vi "Compute Depth Image.vi"() -> ()   [LabVIEW 2014]
doc: "This example demonstrates the binocular stereo vision algorithms installed with NI Vision Development Module."
uses:
  <vilib>/vision/NI_Vision_Development_Module.lvlib
panel:
  out "SGBM Time":dbl caption="Time to Compute Depth Image"
  out "SGBM Time":dbl caption="Time to Compute Depth Image"
  out "SGBM Depth":dbl caption="Depth"
  out "Depth - Block Matching Algorithm":sgl[][](graph)
  out "Depth - Semi Global Block Matching Algorithm":sgl[][](graph)
  out "BM Depth":dbl caption="Depth"
  in  "Stop":bool
  in  "Select Image":i32(slide) min=0 max=5 step=1 scale=0.0..4.0
  out "Calibrating":bool=TRUE
  out "Right Image":T1(plugin-control)
  out "Left Image":T1(plugin-control)
  # "Overview: Demonstrate how to calibrate a stereo vision system and compute a depth image.\nRequirements: Vision Development Module.\nNote: This example does not run on LabVIEW Real Time\nInstructions:\n1. Run the VI.\n2. Select an image with the Select Image control\n3. Mouse over any image to view the depth at the mouse location."
  # "in"
  # "in"
  # "in"
  # "in"
  # "Mouse over the image to view the depth."
  # "inches"
  # "inches"
  # "Mouse over the image to view the depth."
  # "ms"
  # "ms"
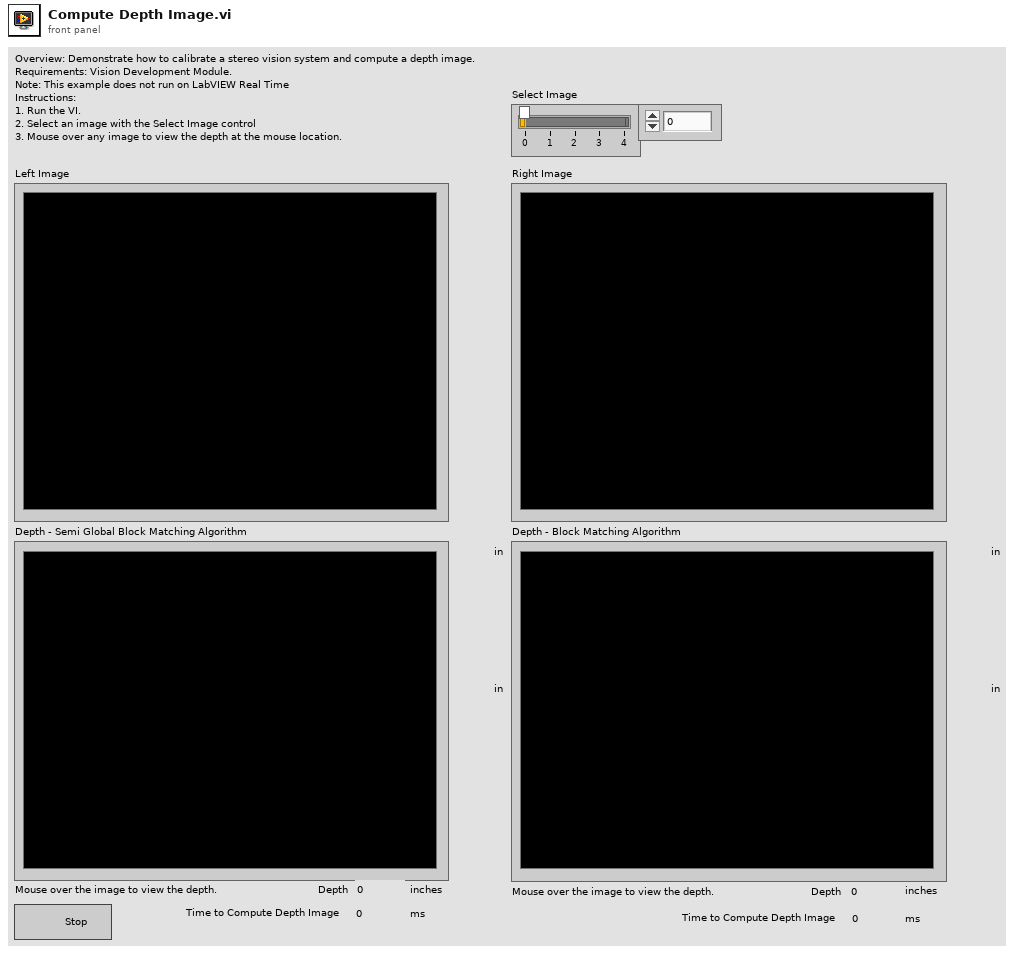
[diagram p1: front panel]
types:
  T1 = typedef "IMAQ Image.ctl" = refnum<image>
  T2 = cluster{"Number of Disparity":dbl, "Number of Disparity":dbl}
  T3 = typedef "Calibration Reference Points.ctl" = cluster{"Pixel Coordinates":cluster{"X":dbl, "Y":dbl}[], "Real World Coordinates":cluster{"X":dbl, "Y":dbl}[], "Unit":T4, "Image Size":cluster{"X":u32, "Y":u32}}
  T4 = typedef "Image Unit" = enum32{"Undefined", "Angström", "Micrometer", "Millimeter", "Centimeter", "Meter", "Kilometer", "Microinch", "Inch", "Feet", "Nautical miles", "Standard miles", "Steps"}
  T5 = typedef "IMAQ Binocular Stereo Session.ctl" = refnum<k1>
  T6 = typedef "Image Type" = u32
  T7 = cluster{"Method":u16, "Window Size":dbl, "Minimum Disparity":dbl, "Number of Disparity":dbl, "Left - Right Check":dbl, "Subpixel":bool, "Invalid Disparity Replace Value":dbl}
  T8 = cluster{"Filter Type":u16, "Filter Size":dbl, "Filter Cap":dbl}
  T9 = cluster{"Texture Threshold":dbl, "Uniqueness Ratio":dbl, "Speckle Window Size":dbl, "Speckle Range":dbl}
  T10 = cluster{"Method":u16, "Window Size":dbl, "Minimum Disparity":dbl, "Number of Disparity":dbl, "P1":dbl, "P2":dbl, "Full DP":bool, "Max Left Right Disparity":dbl, "Subpixel":bool, "Invalid Disparity Replace Value":dbl}
  T11 = typedef "LVPoint32TypeDef.ctl" = cluster{"Horizontal":i32, "Vertical":i32}
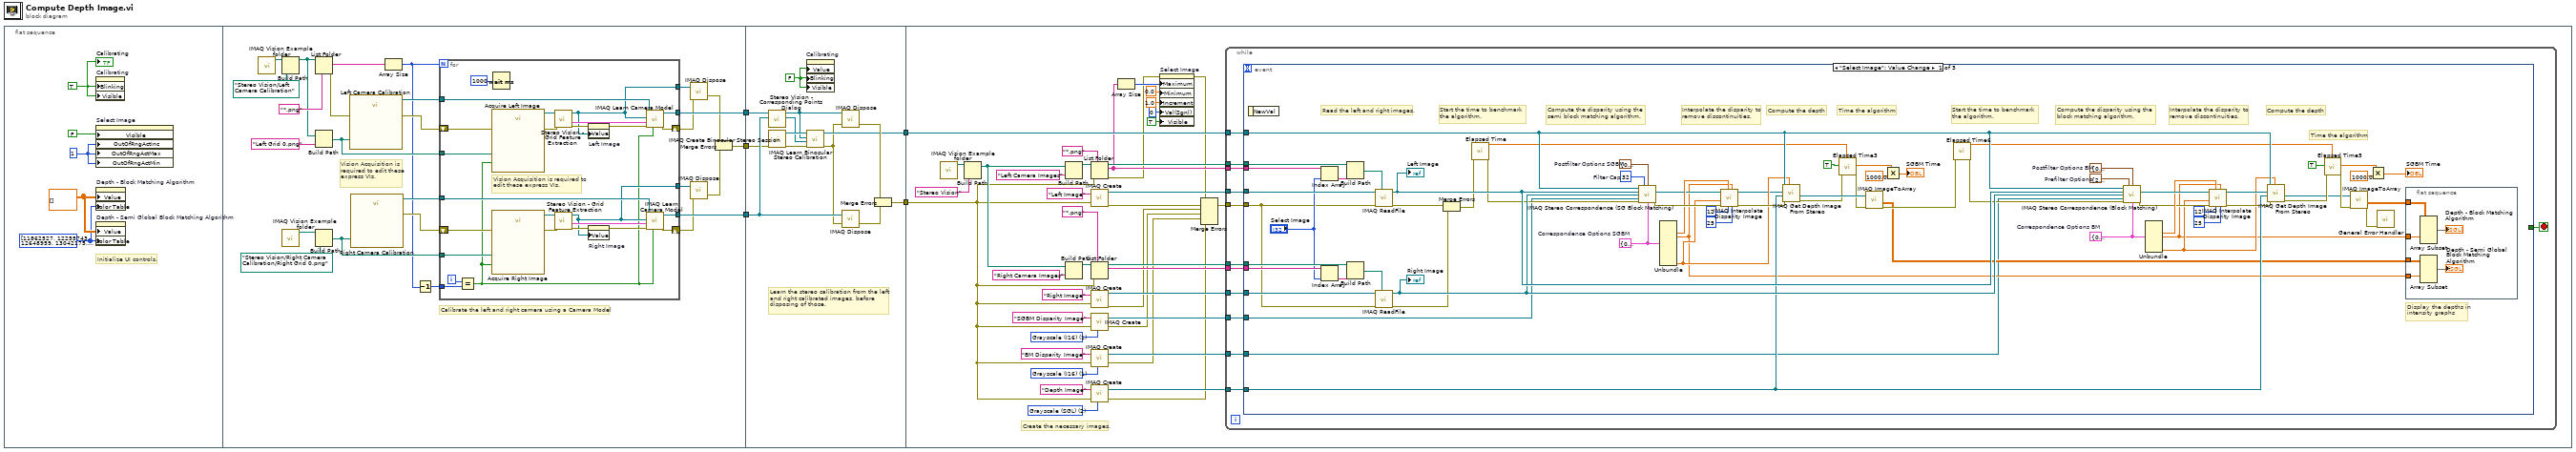
[diagram p0: block diagram]
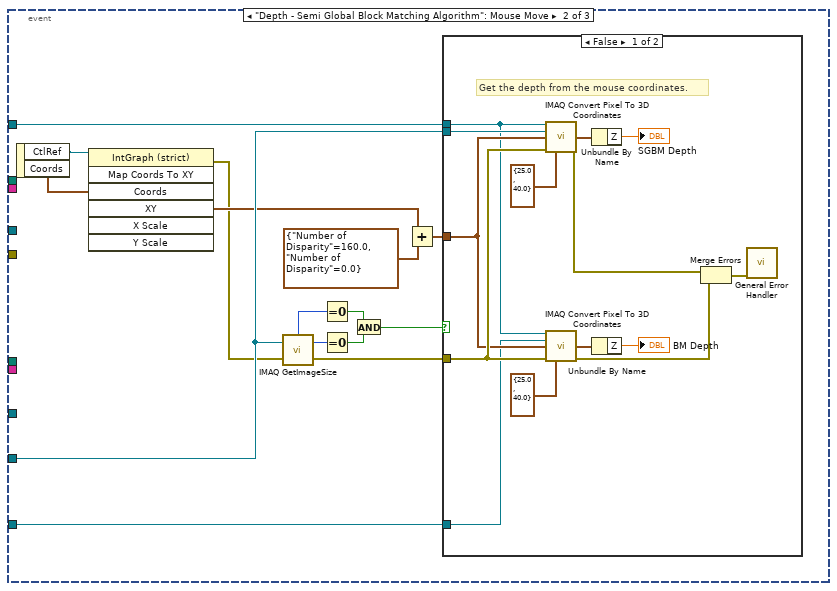
[diagram p2: hidden frame]
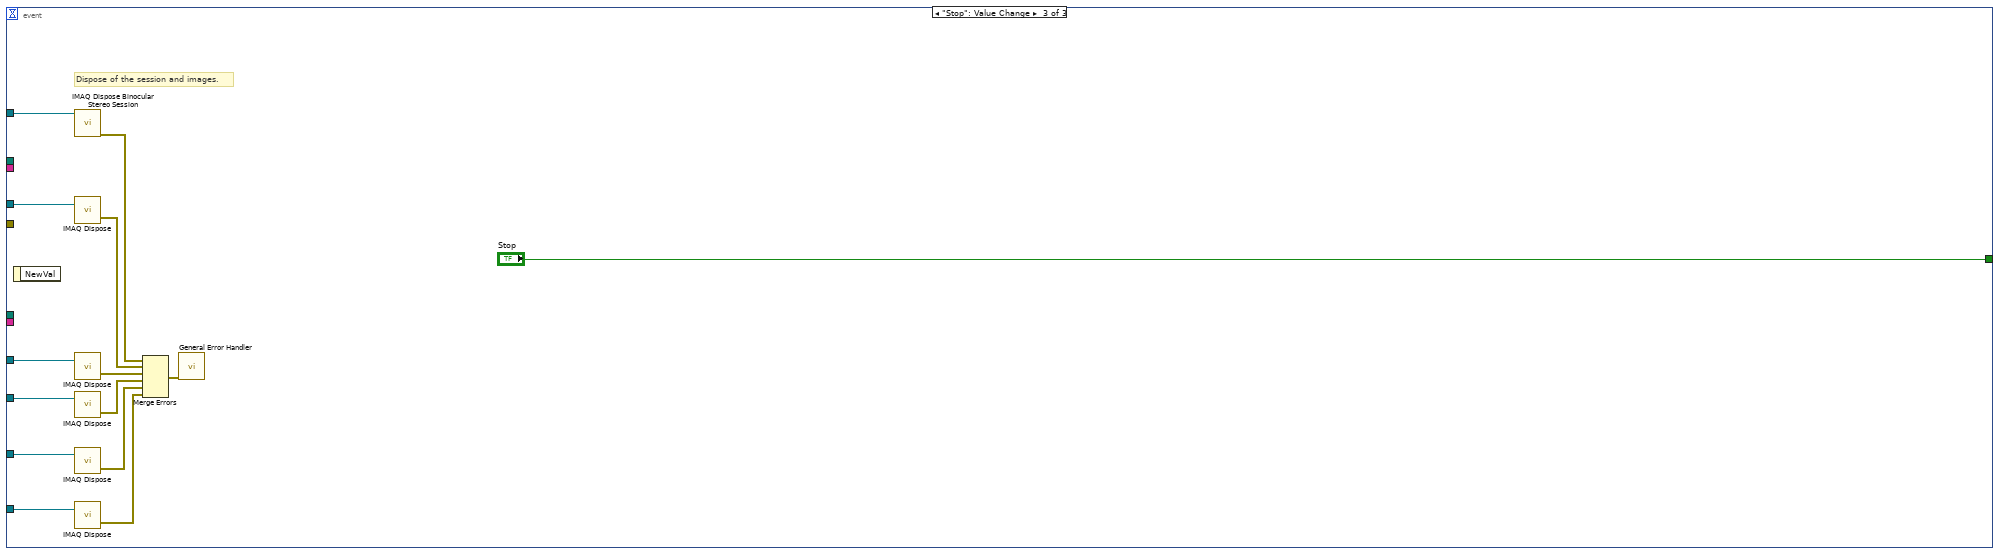
[diagram p4: hidden frame]
diagram:
  n1 = flat-sequence {
    tunnel: [w33] -> w5
    tunnel: [w36] -> w4
    tunnel: [w32] -> w2
    tunnel: w5 -> [w72]
    tunnel: w4 -> [w71]
    tunnel: [w64] -> w3
    tunnel: w2 -> [w68]
    tunnel: [w65] -> w1
    tunnel: w3 -> [w99]
    tunnel: w1 -> [w79]
    frame #0 {
      w6 = u32[] [11862527, 12255743, 12648959, 13042175, 13435391, 13828607, 14221823, 14615039, 15008255, 15401471, 15794687, 16187903, 16581119, 16712189, 16712183, 16712177, 16712171, 16712165, 16712159, 16712153, 16712147, 16712141, 16712135, 16712129, 16712123, 16712117, 16712111, 16712105, 16712099, 16712093, 16712087, 16712081, 16712075, 16712069, 16712063, 16712057, 16712051, 16712045, 16712039, 16712033, 16712027, 16712021, 16712015, 16712009, 16712003, 16711997, 16711991, 16711985, 16711979, 16711973, 16711967, 16711961, 16711955, 16711949, 16711943, 16711937, 16711937, 16713473, 16715009, 16716545, 16718081, 16719617, 16721153, 16722689, 16724225, 16725761, 16727297, 16728833, 16730369, 16731905, 16733441, 16734977, 16736513, 16738049, 16739585, 16741121, 16742657, 16744193, 16745729, 16747265, 16748801, 16750337, 16751873, 16753409, 16754945, 16756481, 16758017, 16759553, 16761089, 16762625, 16765697, 16767233, 16768769, 16770305, 16771841, 16773377, 16774913, 16776449, 16645889, 16252673, 15859457, 15466241, 15073025, 14679809, 14286593, 13893377, 13500161, 13106945, 12713729, 12320513, 11927297, 11534081, 11140865, 10747649, 10354433, 9961217, 9568001, 9174785, 8781569, 8388353, 7995137, 7601921, 7208705, 6815489, 6422273, 6029057, 5635841, 5242625, 4849409, 4456193, 4062977, 3669761, 3276545, 2883329, 2490113, 2096897, 1703681, 1310465, 917249, 524033, 130817, 130823, 130829, 130835, 130841, 130847, 130853, 130859, 130865, 130871, 130877, 130883, 130889, 130895, 130901, 130907, 130913, 130919, 130925, 130931, 130937, 130943, 130949, 130955, 130961, 130967, 130973, 130979, 130985, 130991, 130997, 131003, 131009, 131015, 131021, 131027, 131033, 131039, 131045, 131051, 131057, 131063, 131069, 130559, 129023, 127487, 125951, 124415, 122879, 121343, 119807, 118271, 116735, 115199, 113663, 112127, 110591, 109055, 107519, 105983, 104447, 102911, 101375, 99839, 98303, 96767, 95231, 93695, 92159, 90623, 89087, 87551, 86015, 84479, 82943, 81407, 79871, 78335, 76799, 75263, 255, 248, 240, 233, 226, 219, 211, 204, 197, 189, 182, 175, 168, 160, 153, 146, 138, 131, 124, 117, 109, 102, 95, 87, 80, 73, 66, 58, 51, 44, 36, 29, 22, 15, 7, 0] ("reversed array")
      w7 = sgl[][] [] ("Image")
      w8 = u8 1 ("Response to Value Outside Limits:Maximum")
      w9 = TRUE ("Calibrating")
      # "Initialize UI controls."
      n2 = property on="Calibrating" class="Bool (strict)"("Blinking"=w9, "Visible"=w9) -> ()  [unwired: 2 in, 2 out]
      n3 = property on="Select Image" class="Slide (strict)"("Visible"=FALSE, "OutOfRngActInc"=w8, "OutOfRngActMax"=w8, "OutOfRngActMin"=w8) -> ()  [unwired: 2 in, 2 out]
      n4 = property on="Depth - Block Matching Algorithm" class="IntGraph (strict)"("Value"=w7, "Color Table"=w6) -> ()  [unwired: 2 in, 2 out]
      n5 = property on="Depth - Semi Global Block Matching Algorithm" class="IntGraph (strict)"("Value"=w7, "Color Table"=w6) -> ()  [unwired: 2 in, 2 out]
      "Calibrating" <- w9
    }
    frame #1 {
      # "Vision Acquisition is required to edit these express VIs."
      # "Calibrate the left and right camera using a Camera Model"
      n6 = call "IMAQ Vision Example folder.vi"() -> ("Example Image Path"=w34:path)  [unwired: 11 in]
      n7 = Build Path(base path=w34, name or relative path=path "Stereo Vision/Left Camera Calibration" ("appended path")) -> (appended path=w29:path)
      n8 = call "IMAQ Vision Example folder.vi"() -> ("Example Image Path"=w24:path)  [unwired: 11 in]
      n9 = List Folder(path=w29, pattern="*.png") -> (filenames=w31:string[], error out=w22:errorcluster)  [unwired: 1 in, 3 out]
      n10 = Build Path(base path=w29, name or relative path="Left Grid 0.png" ("pattern")) -> (appended path=w26:path)
      n11 = Build Path(base path=w24, name or relative path=path "Stereo Vision/Right Camera Calibration/Right Grid 0.png" ("appended path")) -> (appended path=w16:path)
      n12 = call "Left Camera Calibration"("Image Path"=w26, "error in"=w22) -> ("Image Out"=w27:T1, "error out"=w21:errorcluster)  [unwired: 24 in]
      n13 = call "Right Camera Calibration"("Image Path"=w16) -> ("Image Out"=w23:T1, "error out"=w20:errorcluster)  [unwired: 25 in]
      n14 = Array Size(array=w31) -> (size(s)=w11:i32)
      n15 = Decrement(x=w11) -> (x-1=w19:i32)
      n16 = for {
        N: w11 -> [_]
        tunnel: w27 -> [w45]
        tunnel: [w62] -> w33
        tunnel: [w52] -> w36
        tunnel: w23 -> [w43]
        tunnel: w19 -> [w61]
        tunnel: w26 -> [w44]
        tunnel: w16 -> [w42]
        tunnel: [w41] -> w18
        tunnel: [w40] -> w17
        shift-right: [w39] -> w15
        shift-left: w21 -> [w50]
        shift-right: [w38] -> w14
        shift-left: w20 -> [w49]
        i -> [w60]
        # "Vision Acquisition is required to edit these express VIs."
        n17 = Equal?(x=w60, y=w61) -> (x = y?=w37:bool)
        n18 = call "Acquire Left Image"("Image Path"=w44, "Stop (F)"=w37, "error in"=w50) -> ("Image Out"=w51:T1, "error out"=w47:errorcluster)  [unwired: 22 in, 1 out]
        n19 = call "Acquire Right Image"("Image Path"=w42, "Stop (F)"=w37, "error in"=w49) -> ("Image Out"=w48:T1, "error out"=w46:errorcluster)  [unwired: 22 in, 1 out]
        n20 = Wait (ms)(milliseconds to wait=u32 1000 ("millisecond timer value")) -> ()  [unwired: 1 out]
        n21 = call "Stereo Vision - Grid Feature Extraction.vi"("error in (no error)"=w47, "Image in"=w51) -> ("error out"=w56:errorcluster, "Reference Points"=w59:T3, "Image (dup)"=w40:T1)  [unwired: 7 out]
        n22 = call "Stereo Vision - Grid Feature Extraction.vi"("error in (no error)"=w46, "Image in"=w48) -> ("error out"=w54:errorcluster, "Reference Points"=w58:T3, "Image (dup)"=w41:T1)  [unwired: 7 out]
        n23 = property on="Left Image" class="ImageControl"(error in=w56, "Value"=w40) -> (error out=w55:errorcluster)  [unwired: 1 in, 1 out]
        n24 = property on="Right Image" class="ImageControl"(error in=w54, "Value"=w41) -> (error out=w53:errorcluster)  [unwired: 1 in, 1 out]
        n25 = call "IMAQ Learn Camera Model"("Add Points and Learn (True)"=w37, "error in (no error)"=w55, "Reference Points"=w59, "Image"=w40, "Calibration Template Image"=w45) -> ("error out"=w39:errorcluster, "Calibration Template Image Out"=w62:T1)  [unwired: 1 in, 4 out]
        n26 = call "IMAQ Learn Camera Model"("Add Points and Learn (True)"=w37, "error in (no error)"=w53, "Reference Points"=w58, "Image"=w41, "Calibration Template Image"=w43) -> ("error out"=w38:errorcluster, "Calibration Template Image Out"=w52:T1)  [unwired: 1 in, 4 out]
      }
      n27 = call "IMAQ Dispose"("Image"=w17, "error in (no error)"=w15) -> ("error out"=w13:errorcluster)  [unwired: 1 in, 3 out]
      n28 = call "IMAQ Dispose"("Image"=w18, "error in (no error)"=w14) -> ("error out"=w12:errorcluster)  [unwired: 1 in, 3 out]
      n29 = Merge Errors(w13, w12) -> (w32:errorcluster)
    }
    frame #2 {
      w75 = FALSE ("Calibrating")
      # "Learn the stereo calibration from the left and right calibrated images, before disposing of those."
      n30 = call "Stereo Vision - Corresponding Points Dialog.vi"("Right Image in"=w71, "Left Image in"=w72) -> ("Right Image out"=w70:T1, "Left Image out"=w69:T1)  [unwired: 7 in, 1 out]
      n31 = call "IMAQ Create Binocular Stereo Session"("error in (no error)"=w68) -> ("error out"=w74:errorcluster, "Binocular Stereo Session Out"=w73:T5)  [unwired: 9 out]
      n32 = property on="Calibrating" class="Bool (strict)"("Value"=w75, "Blinking"=w75, "Visible"=w75) -> ()  [unwired: 2 in, 2 out]
      n33 = call "IMAQ Learn Binocular Stereo Calibration"("error in (no error)"=w74, "Right Calibration Template"=w70, "Left Calibration Template"=w69, "Binocular Stereo Session"=w73) -> ("error out"=w63:errorcluster, "Binocular Stereo Session (dup)"=w64:T5)  [unwired: 1 in, 5 out]
      n34 = call "IMAQ Dispose"("Image"=w69, "error in (no error)"=w63) -> ("error out"=w67:errorcluster)  [unwired: 1 in, 3 out]
      n35 = call "IMAQ Dispose"("Image"=w71, "error in (no error)"=w63) -> ("error out"=w66:errorcluster)  [unwired: 1 in, 3 out]
      n36 = Merge Errors(w67, w66) -> (w65:errorcluster)
    }
    frame #3 {
      w81 = T6 1 items=["Grayscale (U8)", "Grayscale (I16)", "Grayscale (SGL)", "Complex (CSG)", "RGB (U32)", "HSL (U32)", "RGB (U64)", "Grayscale (U16)"] ("Image Type")
      w100 = T6 2 items=["Grayscale (U8)", "Grayscale (I16)", "Grayscale (SGL)", "Complex (CSG)", "RGB (U32)", "HSL (U32)", "RGB (U64)", "Grayscale (U16)"] ("Image Type")
      w101 = T6 1 items=["Grayscale (U8)", "Grayscale (I16)", "Grayscale (SGL)", "Complex (CSG)", "RGB (U32)", "HSL (U32)", "RGB (U64)", "Grayscale (U16)"] ("Image Type")
      # "Create the necessary images."
      n37 = call "IMAQ Vision Example folder.vi"() -> ("Example Image Path"=w95:path)  [unwired: 11 in]
      n38 = Build Path(base path=w95, name or relative path="Stereo Vision") -> (appended path=w94:path)
      n39 = Build Path(base path=w94, name or relative path="Left Camera Images") -> (appended path=w116:path)
      n40 = Build Path(base path=w94, name or relative path="Right Camera Images") -> (appended path=w113:path)
      n41 = List Folder(path=w116, pattern="*.png", error in=w79) -> (path out=w111:path, filenames=w91:string[], error out=w89:errorcluster)  [unwired: 2 out]
      n42 = call "IMAQ Create"("Image Name"="Left Image", "error in (no error)"=w79) -> ("New Image"=w109:T1, "error out"=w87:errorcluster)  [unwired: 2 in, 1 out]
      n43 = List Folder(path=w113, pattern="*.png", error in=w79) -> (path out=w110:path, filenames=w112:string[])  [unwired: 3 out]
      n44 = call "IMAQ Create"("Image Name"="Right Image", "error in (no error)"=w79) -> ("New Image"=w106:T1, "error out"=w85:errorcluster)  [unwired: 2 in, 1 out]
      n45 = call "IMAQ Create"("Image Name"="SGBM Disparity Image", "Image Type"=w101, "error in (no error)"=w79) -> ("New Image"=w104:T1, "error out"=w84:errorcluster)  [unwired: 1 in, 1 out]
      n46 = call "IMAQ Create"("Image Name"="BM Disparity Image", "Image Type"=w81, "error in (no error)"=w79) -> ("New Image"=w78:T1, "error out"=w77:errorcluster)  [unwired: 1 in, 1 out]
      n47 = call "IMAQ Create"("Image Name"="Depth Image", "Image Type"=w100, "error in (no error)"=w79) -> ("New Image"=w102:T1, "error out"=w76:errorcluster)  [unwired: 1 in, 1 out]
      n48 = Array Size(array=w91) -> (size(s)=w90:i32)
      n49 = property on="Select Image" class="Slide (strict)"(error in=w89, "Maximum"=w90, "Minimum"=0.0 ("Data Entry Limits:Minimum"), "Increment"=1.0 ("Data Entry Limits:Increment"), "Val(Sgnl)"=0 ("Value (Signaling)"), "Visible"=TRUE) -> (error out=w88:errorcluster)  [unwired: 1 in, 1 out]
      n50 = Merge Errors(w88, w87, w85, w84, w77, w76) -> (w86:errorcluster)
      n51 = while {
        tunnel: w91 -> [w128]
        tunnel: w112 -> [w127]
        tunnel: w111 -> [w126]
        tunnel: w110 -> [w125]
        tunnel: w109 -> [w124]
        tunnel: w99 -> [w123]
        tunnel: w106 -> [w122]
        tunnel: w104 -> [w121]
        tunnel: w102 -> [w120]
        tunnel: w86 -> [w118]
        tunnel: w78 -> [w117]
        stop <- w119 stop-if-true
        n52 = event shown="[0] \"Select Image\": Value Change" {
          selector: _ -> [_ _ _]
          dyn-events: _ -> [_ _ _]
          timeout: _ -> [_ _ _]
          tunnel: w128 -> [w194 _ _]
          tunnel: w127 -> [w192 _ _]
          tunnel: w126 -> [w195 _ _]
          tunnel: w125 -> [w193 _ _]
          tunnel: w124 -> [w191 _ w243]
          tunnel: w123 -> [w188 w216 w239]
          tunnel: w122 -> [w190 _ w242]
          tunnel: w121 -> [w136 w215 w241]
          tunnel: w120 -> [w185 _ w240]
          tunnel: [_ _ "Stop"] -> w119
          tunnel: w118 -> [w138 _ _]
          tunnel: w117 -> [w137 w202 w238]
          event "Select Image": Value Change {
            w145 = T7 {"Method"=0, "Window Size"=25.0, "Minimum Disparity"=0.0, "Number of Disparity"=160.0, "Left - Right Check"=5.0, "Subpixel"=TRUE, "Invalid Disparity Replace Value"=-16.0}  # Correspondence Options BM
            w146 = T8 {"Filter Type"=2, "Filter Size"=11.0, "Filter Cap"=31.0}  # Prefilter Options
            w147 = T9 {"Texture Threshold"=0.0, "Uniqueness Ratio"=0.0, "Speckle Window Size"=5.0, "Speckle Range"=200.0}  # Postfilter Options BM
            w167 = T10 {"Method"=0, "Window Size"=25.0, "Minimum Disparity"=0.0, "Number of Disparity"=160.0, "P1"=100.0, "P2"=500.0, "Full DP"=FALSE, "Max Left Right Disparity"=5.0, "Subpixel"=TRUE, "Invalid Disparity Replace Value"=-16.0}  # Correspondence Options SGBM
            w165 = u32 32  # Filter Cap
            w166 = T9 {"Texture Threshold"=0.0, "Uniqueness Ratio"=0.0, "Speckle Window Size"=5.0, "Speckle Range"=200.0}  # Postfilter Options SGBM
            # "Time the algorithm"
            # "Interpolate the disparity to remove discontinuities."
            # "Start the time to benchmark the algorithm."
            # "Time the algorithm"
            # "Start the time to benchmark the algorithm."
            # "Display the depths in intensity graphs"
            # "Compute the depth"
            # "Compute the disparity using the block matching algorithm."
            # "Compute the depth"
            # "Interpolate the disparity to remove discontinuities."
            # "Compute the disparity using the semi block matching algorithm."
            # "Read the left and right images."
            n53 = event-data() -> ()  [unwired: 2 out]
            n54 = Index Array(array=w194, index="Select Image") -> (element=w182:string)
            n55 = Index Array(array=w192, index="Select Image") -> (element=w181:string)
            n56 = Build Path(base path=w195, name or relative path=w182) -> (appended path=w180:path)
            n57 = Build Path(base path=w193, name or relative path=w181) -> (appended path=w178:path)
            n58 = call "IMAQ ReadFile"("File Path"=w180, "error in (no error)"=w138, "Image"=w191) -> ("error out"=w183:errorcluster, "Image Out"=w187:T1)  [unwired: 2 in, 5 out]
            "Left Image" <- w187
            n59 = call "IMAQ ReadFile"("File Path"=w178, "error in (no error)"=w138, "Image"=w190) -> ("error out"=w184:errorcluster, "Image Out"=w186:T1)  [unwired: 2 in, 5 out]
            "Right Image" <- w186
            n60 = Merge Errors(w183, w184) -> (w160:errorcluster)
            n61 = call "Elapsed Time"("error in (no error)"=w160) -> ("Present (s)"=w175:dbl, "error out"=w164:errorcluster)  [unwired: 11 in, 6 out]
            n62 = call "IMAQ Stereo Correspondence (SG Block Matching)"("Binocular Stereo Session"=w188, "Filter Cap"=w165, "Postfilter Options"=w166, "Left Image In"=w187, "Right Image In"=w186, "Disparity Image In"=w136, "error in (no error)"=w164, "Correspondence Options"=w167) -> ("Disparity Image Out"=w168:T1, "error out"=w172:errorcluster)  [unwired: 2 in, 4 out]
            n63 = Unbundle(w167) -> ("Minimum Disparity"=w169:dbl, "Number of Disparity"=w162:dbl, "Invalid Disparity Replace Value"=w171:dbl)  [unwired: 7 out]
            n64 = call "IMAQ Interpolate Disparity Image"("Sampling Frequency"=25, "Number of Disparities"=w162, "Order"=12, "Minimum Disparity"=w169, "error in (no error)"=w172, "Invalid Disparity Value"=w171, "Image Src"=w168) -> ("error out"=w173:errorcluster, "Image Dst Out"=w170:T1)  [unwired: 1 in, 2 out]
            n65 = call "IMAQ Get Depth Image From Stereo"("Invalid Disparity Value"=w171, "error in (no error)"=w173, "Depth Image In"=w185, "Disparity Image"=w170, "Binocular Stereo Session"=w188) -> ("error out"=w174:errorcluster, "Depth Image Out"=w177:T1)  [unwired: 2 in, 3 out]
            n66 = call "Elapsed Time3"("Reset"=TRUE, "error in (no error)"=w174, "Set Start Time (s)"=w175) -> ("Elapsed Time (s)"=w133:dbl, "error out"=w176:errorcluster)  [unwired: 9 in, 6 out]
            n67 = call "IMAQ ImageToArray"("error in (no error)"=w176, "Image"=w177) -> ("Image Pixels (Float)"=w163:sgl[][], "error out"=w189:errorcluster)  [unwired: 1 in, 4 out]
            n68 = Multiply(x=w133, y=1000.0) -> (x*y=→"SGBM Time":dbl)
            n69 = call "Elapsed Time6"("error in (no error)"=w189) -> ("Present (s)"=w150:dbl, "error out"=w157:errorcluster)  [unwired: 11 in, 6 out]
            n70 = call "IMAQ Stereo Correspondence (Block Matching)"("Binocular Stereo Session"=w188, "Prefilter Options"=w146, "Postfilter Options"=w147, "Left Image In"=w187, "Right Image In"=w186, "Disparity Image In"=w137, "error in (no error)"=w157, "Correspondence Options"=w145) -> ("Disparity Image Out"=w156:T1, "error out"=w153:errorcluster)  [unwired: 4 in, 2 out]
            n71 = Unbundle(w145) -> ("Minimum Disparity"=w155:dbl, "Number of Disparity"=w142:dbl, "Invalid Disparity Replace Value"=w144:dbl)  [unwired: 4 out]
            n72 = call "IMAQ Interpolate Disparity Image"("Sampling Frequency"=25, "Number of Disparities"=w142, "Order"=12, "Minimum Disparity"=w155, "error in (no error)"=w153, "Invalid Disparity Value"=w144, "Image Src"=w156) -> ("error out"=w152:errorcluster, "Image Dst Out"=w154:T1)  [unwired: 1 in, 2 out]
            n73 = call "IMAQ Get Depth Image From Stereo"("Invalid Disparity Value"=w144, "error in (no error)"=w152, "Depth Image In"=w185, "Disparity Image"=w154, "Binocular Stereo Session"=w188) -> ("error out"=w151:errorcluster, "Depth Image Out"=w148:T1)  [unwired: 2 in, 3 out]
            n74 = call "Elapsed Time5"("Reset"=TRUE, "error in (no error)"=w151, "Set Start Time (s)"=w150) -> ("Elapsed Time (s)"=w130:dbl, "error out"=w149:errorcluster)  [unwired: 9 in, 6 out]
            n75 = call "IMAQ ImageToArray"("error in (no error)"=w149, "Image"=w148) -> ("Image Pixels (Float)"=w143:sgl[][], "error out"=w135:errorcluster)  [unwired: 1 in, 4 out]
            n76 = Multiply(x=w130, y=1000.0) -> (x*y=→"SGBM Time":dbl)
            n77 = call <vilib>:"General Error Handler.vi"("error in (no error)"=w135) -> ()  [unwired: 10 in, 5 out]
            n78 = flat-sequence {
              tunnel: w163 -> [w201]
              tunnel: w162 -> [w200]
              tunnel: w143 -> [w198]
              tunnel: w142 -> [w197]
              frame #0 {
                n79 = Array Subset(array=w198, index (col)=w197) -> (→"Depth - Block Matching Algorithm":sgl[][])  [unwired: 3 in]
                n80 = Array Subset(array=w201, index (col)=w200) -> (→"Depth - Semi Global Block Matching Algorithm":sgl[][])  [unwired: 3 in]
              }
            }
          }
          event "Depth - Semi Global Block Matching Algorithm": Mouse Move {
            n81 = event-data() -> ("CtlRef"=w207:refnum<vi>, "Coords"=w206:T11)  [unwired: 1 out]
            n82 = invoke class="IntGraph (strict)" method="Map Coords To XY"(reference=w207, "Coords"=w206) -> (error out=w204:errorcluster, "XY"=w209:cluster{"X":dbl, "Y":dbl})  [unwired: 5 in, 5 out]
            n83 = call "IMAQ GetImageSize"("Image"=w215, "error in (no error)"=w204) -> ("Y Resolution"=w213:i32, "X Resolution"=w214:i32, "error out"=w203:errorcluster)  [unwired: 2 out]
            n84 = Equal To 0?(x=w214) -> (x = 0?=w212:bool)
            n85 = Equal To 0?(x=w213) -> (x = 0?=w211:bool)
            n86 = And(x=w212, y=w211) -> (x .and. y?=w210:bool)
            n87 = Add(x=w209, y=T2 {"Number of Disparity"=160.0, "Number of Disparity"=0.0} ("output cluster")) -> (x+y=w208:cluster{dbl, dbl})
            n88 = case shown="False" w210 {
              tunnel: w216 -> [w221 _]
              tunnel: w215 -> [w230 _]
              tunnel: w208 -> [w222 _]
              tunnel: w203 -> [w224 _]
              tunnel: w202 -> [w220 _]
              frame False {
                # "Get the depth from the mouse coordinates."
                n89 = call "IMAQ Convert Pixel To 3D Coordinates"("Binocular Stereo Session"=w221, "Disparity Image"=w230, "Pixel Coordinates"=w222, "error in (no error)"=w224, "Depth Control"=cluster{"Min Depth":dbl, "Max Depth":dbl} {"Min Depth"=25.0, "Max Depth"=40.0}) -> ("Real World 3D Coordinates"=w229:cluster{"X":dbl, "Y":dbl, "Z":dbl}, "error out"=w219:errorcluster)  [unwired: 3 in, 6 out]
                n90 = call "IMAQ Convert Pixel To 3D Coordinates"("Binocular Stereo Session"=w221, "Disparity Image"=w220, "Pixel Coordinates"=w222, "error in (no error)"=w224, "Depth Control"=cluster{"Min Depth":dbl, "Max Depth":dbl} {"Min Depth"=25.0, "Max Depth"=40.0}) -> ("Real World 3D Coordinates"=w225:cluster{"X":dbl, "Y":dbl, "Z":dbl}, "error out"=w218:errorcluster)  [unwired: 3 in, 6 out]
                n91 = Unbundle By Name(w229) -> ("Z"=→"SGBM Depth":dbl)
                n92 = Unbundle By Name(w225) -> ("Z"=→"BM Depth":dbl)
                n93 = Merge Errors(w219, w218) -> (w217:errorcluster)
                n94 = call <vilib>:"General Error Handler.vi"("error in (no error)"=w217) -> ()  [unwired: 10 in, 5 out]
              }
              frame True {
              }
            }
          }
          event "Stop": Value Change {
            # "Dispose of the session and images."
            n95 = event-data() -> ()  [unwired: 2 out]
            n96 = call "IMAQ Dispose Binocular Stereo Session"("Binocular Stereo Session"=w239) -> ("error out"=w236:errorcluster)  [unwired: 1 in, 9 out]
            n97 = call "IMAQ Dispose"("Image"=w243) -> ("error out"=w235:errorcluster)  [unwired: 2 in, 3 out]
            n98 = call "IMAQ Dispose"("Image"=w242) -> ("error out"=w234:errorcluster)  [unwired: 2 in, 3 out]
            n99 = call "IMAQ Dispose"("Image"=w241) -> ("error out"=w233:errorcluster)  [unwired: 2 in, 3 out]
            n100 = call "IMAQ Dispose"("Image"=w238) -> ("error out"=w232:errorcluster)  [unwired: 2 in, 3 out]
            n101 = call "IMAQ Dispose"("Image"=w240) -> ("error out"=w231:errorcluster)  [unwired: 2 in, 3 out]
            n102 = Merge Errors(w236, w235, w234, w233, w232, w231) -> (w237:errorcluster)
            n103 = call <vilib>:"General Error Handler.vi"("error in (no error)"=w237) -> ()  [unwired: 10 in, 5 out]
          }
        }
      }
    }
  }
